vi "DSF.Shared.Configuration.Transfer.Get Access Mode.vi"(8 "error in (no error)":errorcluster, 11 "Transfer Configuration in":refnum<class "DSF.Shared.Configuration.Transfer.lvclass">) -> (0 "error out":errorcluster, 2 "Access":T1=enum."Write", 3 "Transfer Configuration out":refnum<class "DSF.Shared.Configuration.Transfer.lvclass">)   [LabVIEW 2016, in "DSF.Shared.lvlib" / "DSF.Shared.Configuration.Transfer.lvclass"]
uses:
  DSF.Shared.Configuration.Transfer.lvclass
  <vilib>/NI Veristand/Custom Device API/Data Access Type.ctl
  DSF.Shared.Configuration.Transfer.lvclass/DSF.Shared.Configuration.Transfer.ctl
  <vilib>/NI Veristand/Custom Device API/Custom Device API.lvlib
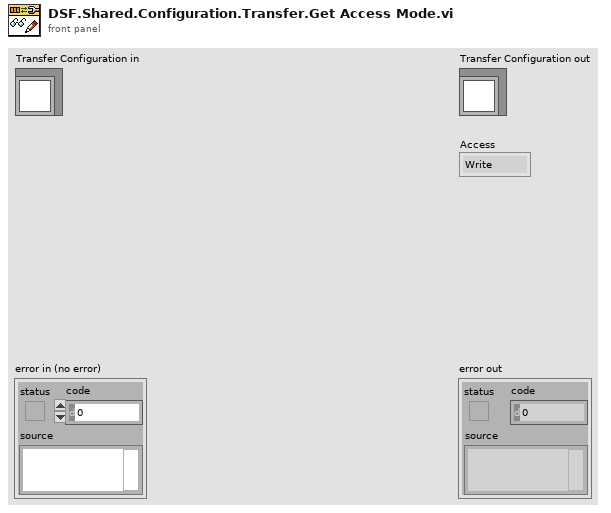
[diagram p1: front panel]
types:
  T1 = typedef "Custom Device API.lvlib/Data Access Type.ctl" = enum16{"Read", "Write"}
  T2 = typedef "DSF.Shared.lvlib/DSF.Shared.Typedefs.Direction.ctl" = enum16{"Tx", "Rx"}
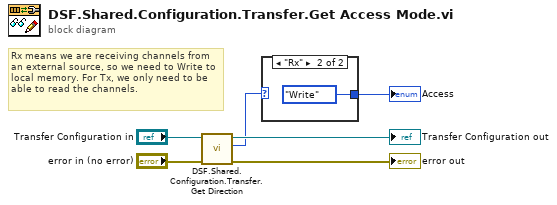
[diagram p0: block diagram]
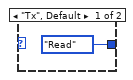
[diagram p2: hidden frame]
diagram:
  # "Rx means we are receiving channels from an external source, so we need to Write to local memory. For Tx, we only need to be able to read the channels."
  n1 = call "DSF.Shared.Configuration.Transfer.Get Direction.vi"("error in (no error)"="error in (no error)", "Transfer Configuration in"="Transfer Configuration in") -> ("error out"=→"error out":errorcluster, "Direction"=w1:T2, "Transfer Configuration out"=→"Transfer Configuration out":refnum<class "DSF.Shared.Configuration.Transfer.lvclass">)  [unwired: 7 in]
  n2 = case shown="\"Rx\"" w1 {
    tunnel: [Data_Access_Type."Read" ("Access") Data_Access_Type."Write" ("Access")] -> w4
    frame "Tx", Default {
    }
    frame "Rx" {
    }
  }
  "Access" <- w4
